vi "DCC_SplitClusterAndCheck.vi"(6 "Data Cluster":T4, 8 "Error In":errorcluster, 10 "OLD-DCCControlCluster":T1={"Connector 1"={"Gain/HV [%]"=0.0, "+12V"=FALSE, "+5V"=FALSE, "-5V"=FALSE}, "Connector 2"={"+12V"=FALSE, "+5V"=FALSE, "-5V"=FALSE, "DO0"=FALSE, "DO1"=FALSE, "DO2"=FALSE, "DO3"=FALSE, "DO4"=FALSE, "DO5"=FALSE, "DO6"=FALSE, "DO7"=FALSE}, "Connector 3"={"Gain/HV [%]"=0.0, "+12V"=FALSE, "+5V"=FALSE, "-5V"=FALSE}, "Cooler Current [A]"=0.0, "Cooler Volt [V]"=0.0, "Cooling"=FALSE, "Enable Outputs"=FALSE, "AutoGain1"=FALSE, "AutoGain3"=FALSE, "Current Limit"=FALSE, "Overload"=FALSE, "LabelCon1"="Connector 1", "LabelCon2"="Connector 2", "LabelCon3"="Connector 3"} {"Cooler Volt [V]" scale=0.0..5.0; "Cooler Current [A]" scale=0.0..2.0; "Connector 3"."Gain/HV [%]" scale=0.0..100.0; "Connector 1"."Gain/HV [%]" scale=0.0..100.0}, 11 "NEW-DCCControlCluster":T1={"Connector 1"={"Gain/HV [%]"=0.0, "+12V"=FALSE, "+5V"=FALSE, "-5V"=FALSE}, "Connector 2"={"+12V"=FALSE, "+5V"=FALSE, "-5V"=FALSE, "DO0"=FALSE, "DO1"=FALSE, "DO2"=FALSE, "DO3"=FALSE, "DO4"=FALSE, "DO5"=FALSE, "DO6"=FALSE, "DO7"=FALSE}, "Connector 3"={"Gain/HV [%]"=0.0, "+12V"=FALSE, "+5V"=FALSE, "-5V"=FALSE}, "Cooler Current [A]"=0.0, "Cooler Volt [V]"=0.0, "Cooling"=FALSE, "Enable Outputs"=FALSE, "AutoGain1"=FALSE, "AutoGain3"=FALSE, "Current Limit"=FALSE, "Overload"=FALSE, "LabelCon1"="Connector 1", "LabelCon2"="Connector 2", "LabelCon3"="Connector 3"} {"Cooler Volt [V]" scale=0.0..5.0; "Cooler Current [A]" scale=0.0..2.0; "Connector 3"."Gain/HV [%]" scale=0.0..100.0; "Connector 1"."Gain/HV [%]" scale=0.0..100.0}) -> (0 "Error Out":errorcluster, 2 "Unequal To\nPrevious?":bool, 4 "Data Cluster":T4)   [LabVIEW 2019]
doc: "This function splits the corresponding cluster to its elements and checks whether there had occured a change in values. \nFurther, just the values will be handled which had changed. If there is a change all current values will be written into the Data Cluster of the SPC module.\n\nOktober 2018\nFrank Quadt & Stefan Smietana\ninfo@becker-hickl.com"
uses:
  DCC_Controls/DCC_ControlCluster.ctl
  DCC_Controls/DCC_Connector1.ctl
  DCC_Controls/DCC_Connector2.ctl
  DCC_Controls/DCC_Data_Cluster.ctl
panel:
  # "(c) 2018 Becker & Hickl GmbH\n     All Rights Reserved."
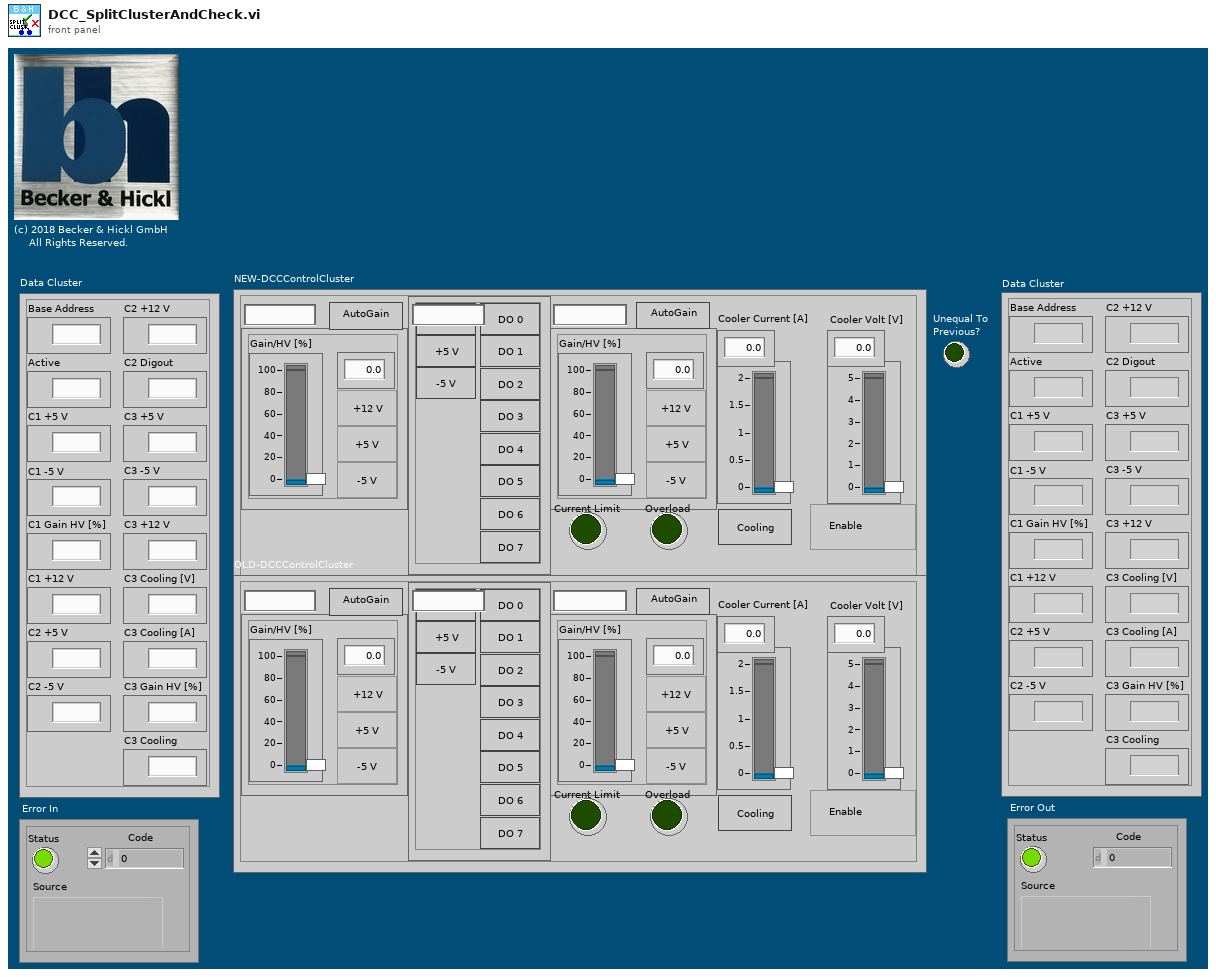
[diagram p1: front panel]
types:
  T1 = typedef "DCC_ControlCluster.ctl" = cluster{"Connector 1":T2, "Connector 2":T3, "Connector 3":T2, "Cooler Current [A]":dbl, "Cooler Volt [V]":dbl, "Cooling":bool, "Enable Outputs":bool, "AutoGain1":bool, "AutoGain3":bool, "Current Limit":bool, "Overload":bool, "LabelCon1":string, "LabelCon2":string, "LabelCon3":string}
  T2 = typedef "DCC_Connector1.ctl" = cluster{"Gain/HV [%]":dbl, "+12V":bool, "+5V":bool, "-5V":bool}
  T3 = typedef "DCC_Connector2.ctl" = cluster{"+12V":bool, "+5V":bool, "-5V":bool, "DO0":bool, "DO1":bool, "DO2":bool, "DO3":bool, "DO4":bool, "DO5":bool, "DO6":bool, "DO7":bool}
  T4 = typedef "DCC_Data_Cluster.ctl" = cluster{"Base Address":u16, "Active":i16, "C1 +5 V":i16, "C1 -5 V":i16, "C1 Gain HV [%]":sgl, "C1 +12 V":i16, "C2 +5 V":i16, "C2 -5 V":i16, "C2 +12 V":i16, "C2 Digout":i16, "C3 +5 V":i16, "C3 -5 V":i16, "C3 +12 V":i16, "C3 Cooling [V]":sgl, "C3 Cooling [A]":sgl, "C3 Gain HV [%]":sgl, "C3 Cooling":i16}
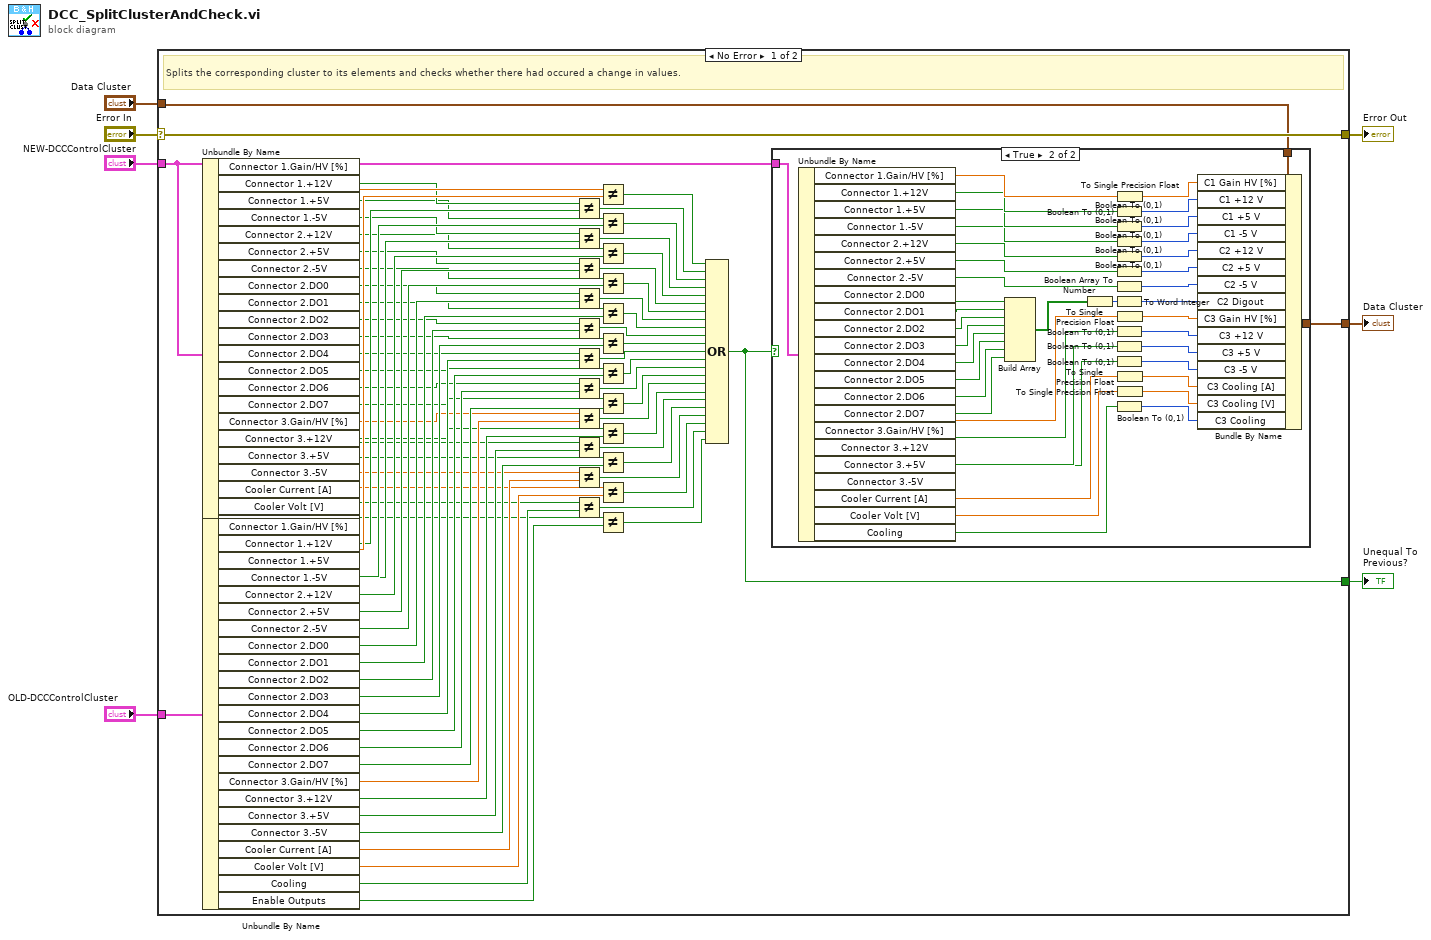
[diagram p0: block diagram]
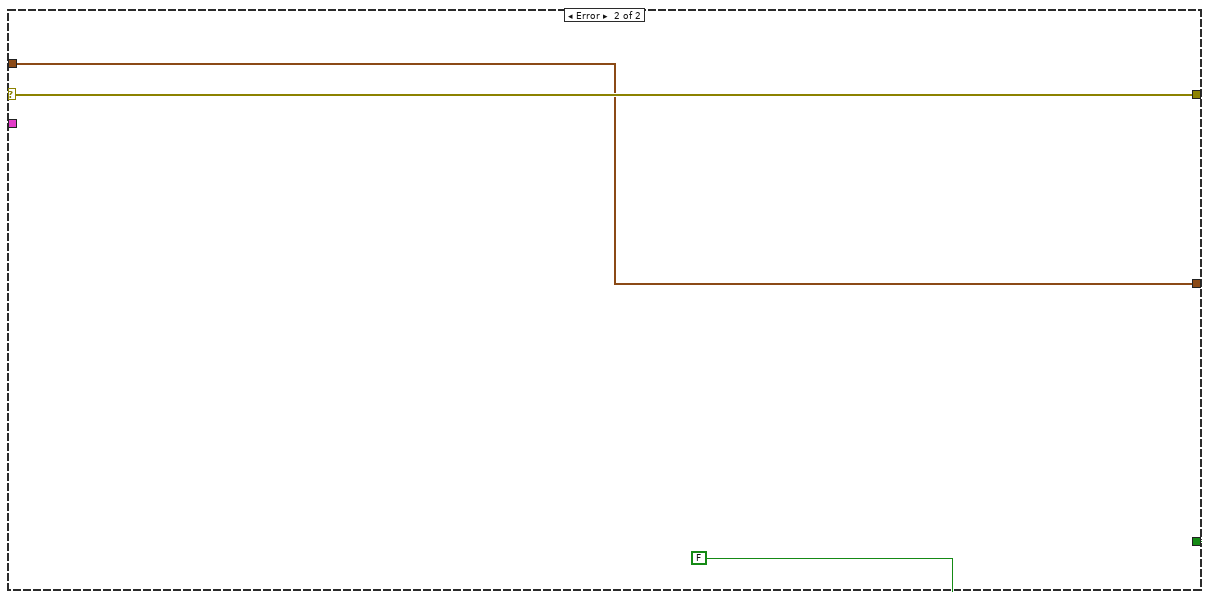
[diagram p3: hidden frame]
diagram:
  n1 = case shown="No Error" "Error In" {
    selector: "Error In" -> [w82 w128]
    tunnel: "NEW-DCCControlCluster" -> [w78 _]
    tunnel: [w8 FALSE] -> w6
    tunnel: [w82 w128] -> w4
    tunnel: "Data Cluster" -> [w81 w126]
    tunnel: [w80 w126] -> w2
    tunnel: "OLD-DCCControlCluster" -> [w79 _]
    frame No Error {
      # "Splits the corresponding cluster to its elements and checks whether there had occured a change in values."
      n2 = Unbundle By Name(w78) -> ("Connector 1.Gain/HV [%]"=w77:dbl, "Connector 1.+12V"=w75:bool, "Connector 1.+5V"=w73:bool, "Connector 1.-5V"=w71:bool, "Connector 2.+12V"=w69:bool, "Connector 2.+5V"=w67:bool, "Connector 2.-5V"=w65:bool, "Connector 2.DO0"=w63:bool, "Connector 2.DO1"=w61:bool, "Connector 2.DO2"=w59:bool, "Connector 2.DO3"=w57:bool, "Connector 2.DO4"=w55:bool, "Connector 2.DO5"=w53:bool, "Connector 2.DO6"=w51:bool, "Connector 2.DO7"=w49:bool, "Connector 3.Gain/HV [%]"=w47:dbl, "Connector 3.+12V"=w45:bool, "Connector 3.+5V"=w43:bool, "Connector 3.-5V"=w41:bool, "Cooler Current [A]"=w39:dbl, "Cooler Volt [V]"=w37:dbl, "Cooling"=w35:bool, "Enable Outputs"=w33:bool)
      n3 = Unbundle By Name(w79) -> ("Connector 1.Gain/HV [%]"=w76:dbl, "Connector 1.+12V"=w74:bool, "Connector 1.+5V"=w72:bool, "Connector 1.-5V"=w70:bool, "Connector 2.+12V"=w68:bool, "Connector 2.+5V"=w66:bool, "Connector 2.-5V"=w64:bool, "Connector 2.DO0"=w62:bool, "Connector 2.DO1"=w60:bool, "Connector 2.DO2"=w58:bool, "Connector 2.DO3"=w56:bool, "Connector 2.DO4"=w54:bool, "Connector 2.DO5"=w52:bool, "Connector 2.DO6"=w50:bool, "Connector 2.DO7"=w48:bool, "Connector 3.Gain/HV [%]"=w46:dbl, "Connector 3.+12V"=w44:bool, "Connector 3.+5V"=w42:bool, "Connector 3.-5V"=w40:bool, "Cooler Current [A]"=w38:dbl, "Cooler Volt [V]"=w36:dbl, "Cooling"=w34:bool, "Enable Outputs"=w32:bool)
      n4 = Not Equal?(x=w75, y=w74) -> (x != y?=w10:bool)
      n5 = Not Equal?(x=w71, y=w70) -> (x != y?=w12:bool)
      n6 = Not Equal?(x=w67, y=w66) -> (x != y?=w14:bool)
      n7 = Not Equal?(x=w63, y=w62) -> (x != y?=w16:bool)
      n8 = Not Equal?(x=w59, y=w58) -> (x != y?=w18:bool)
      n9 = Not Equal?(x=w55, y=w54) -> (x != y?=w30:bool)
      n10 = Not Equal?(x=w51, y=w50) -> (x != y?=w28:bool)
      n11 = Not Equal?(x=w47, y=w46) -> (x != y?=w26:bool)
      n12 = Not Equal?(x=w43, y=w42) -> (x != y?=w24:bool)
      n13 = Not Equal?(x=w39, y=w38) -> (x != y?=w22:bool)
      n14 = Not Equal?(x=w35, y=w34) -> (x != y?=w20:bool)
      n15 = Not Equal?(x=w77, y=w76) -> (x != y?=w9:bool)
      n16 = Not Equal?(x=w73, y=w72) -> (x != y?=w11:bool)
      n17 = Not Equal?(x=w69, y=w68) -> (x != y?=w13:bool)
      n18 = Not Equal?(x=w65, y=w64) -> (x != y?=w15:bool)
      n19 = Not Equal?(x=w61, y=w60) -> (x != y?=w17:bool)
      n20 = Not Equal?(x=w57, y=w56) -> (x != y?=w31:bool)
      n21 = Not Equal?(x=w53, y=w52) -> (x != y?=w29:bool)
      n22 = Not Equal?(x=w49, y=w48) -> (x != y?=w27:bool)
      n23 = Not Equal?(x=w45, y=w44) -> (x != y?=w25:bool)
      n24 = Not Equal?(x=w41, y=w40) -> (x != y?=w23:bool)
      n25 = Not Equal?(x=w37, y=w36) -> (x != y?=w21:bool)
      n26 = Not Equal?(x=w33, y=w32) -> (x != y?=w19:bool)
      n27 = Compound Arithmetic op=OR(w9, w10, w11, w12, w13, w14, w15, w16, w17, w18, w31, w30, w29, w28, w27, w26, w25, w24, w23, w22, w21, w20, w19) -> (w8:bool)
      n28 = case shown="True" w8 {
        tunnel: w81 -> [w83 w123]
        tunnel: w78 -> [_ w125]
        tunnel: [w83 w108] -> w80
        frame False {
        }
        frame True {
          n29 = Unbundle By Name(w125) -> ("Connector 1.Gain/HV [%]"=w122:dbl, "Connector 1.+12V"=w119:bool, "Connector 1.+5V"=w117:bool, "Connector 1.-5V"=w115:bool, "Connector 2.+12V"=w113:bool, "Connector 2.+5V"=w111:bool, "Connector 2.-5V"=w109:bool, "Connector 2.DO0"=w95:bool, "Connector 2.DO1"=w94:bool, "Connector 2.DO2"=w92:bool, "Connector 2.DO3"=w91:bool, "Connector 2.DO4"=w90:bool, "Connector 2.DO5"=w89:bool, "Connector 2.DO6"=w88:bool, "Connector 2.DO7"=w87:bool, "Connector 3.Gain/HV [%]"=w106:dbl, "Connector 3.+12V"=w86:bool, "Connector 3.+5V"=w85:bool, "Connector 3.-5V"=w84:bool, "Cooler Current [A]"=w101:dbl, "Cooler Volt [V]"=w99:dbl, "Cooling"=w97:bool)
          n30 = Build Array(w95, w94, w92, w91, w90, w89, w88, w87) -> (w93:bool[])
          n31 = Boolean Array To Number(Boolean array=w93) -> (number=w124:u32)
          n32 = Boolean To (0,1)(Boolean=w119) -> (0, 1=w120:i16)
          n33 = Boolean To (0,1)(Boolean=w117) -> (0, 1=w118:i16)
          n34 = Boolean To (0,1)(Boolean=w115) -> (0, 1=w116:i16)
          n35 = Boolean To (0,1)(Boolean=w113) -> (0, 1=w114:i16)
          n36 = Boolean To (0,1)(Boolean=w111) -> (0, 1=w112:i16)
          n37 = Boolean To (0,1)(Boolean=w109) -> (0, 1=w110:i16)
          n38 = To Word Integer(number=w124) -> (16bit integer=w96:i16)
          n39 = Boolean To (0,1)(Boolean=w86) -> (0, 1=w105:i16)
          n40 = Boolean To (0,1)(Boolean=w85) -> (0, 1=w104:i16)
          n41 = Boolean To (0,1)(Boolean=w84) -> (0, 1=w103:i16)
          n42 = Boolean To (0,1)(Boolean=w97) -> (0, 1=w98:i16)
          n43 = To Single Precision Float(number=w122) -> (single precision float=w121:sgl)
          n44 = To Single Precision Float(number=w106) -> (single precision float=w107:sgl)
          n45 = To Single Precision Float(number=w101) -> (single precision float=w102:sgl)
          n46 = To Single Precision Float(number=w99) -> (single precision float=w100:sgl)
          n47 = Bundle By Name(cluster=w123, "C1 Gain HV [%]"=w121, "C1 +12 V"=w120, "C1 +5 V"=w118, "C1 -5 V"=w116, "C2 +12 V"=w114, "C2 +5 V"=w112, "C2 -5 V"=w110, "C2 Digout"=w96, "C3 Gain HV [%]"=w107, "C3 +12 V"=w105, "C3 +5 V"=w104, "C3 -5 V"=w103, "C3 Cooling [A]"=w102, "C3 Cooling [V]"=w100, "C3 Cooling"=w98) -> (w108:T4)
        }
      }
    }
    frame Error {
    }
  }
  "Unequal To\nPrevious?" <- w6
  "Error Out" <- w4
  "Data Cluster" <- w2
